vi "Datatype to Datatype String.vi"(11 "Generic Datatype":T1=enum."Bool") -> (2 "Rust String":string, 3 "String":string)   [LabVIEW 2021, in "DataTypes_CIF_U.lvlib"]
doc: "Convert generic datatypes into string names."
uses:
  DataTypes_CIF_U.lvlib
  Typedef/Generic Datatypes.ctl
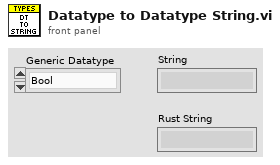
[diagram p1: front panel]
types:
  T1 = typedef "DataTypes_CIF_U.lvlib/Generic Datatypes.ctl" = enum16{"Invalid", "Bool", "U8", "I8", "U16", "I16", "U32", "I32", "U64", "I64", "Single Float", "Double Float", "String"}
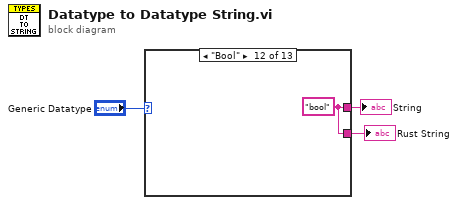
[diagram p0: block diagram]
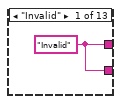
[diagram p2: hidden frame]
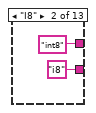
[diagram p3: hidden frame]
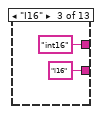
[diagram p4: hidden frame]
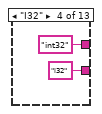
[diagram p5: hidden frame]
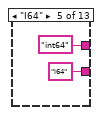
[diagram p6: hidden frame]
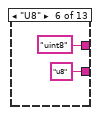
[diagram p7: hidden frame]
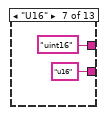
[diagram p8: hidden frame]
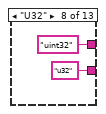
[diagram p9: hidden frame]
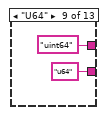
[diagram p10: hidden frame]
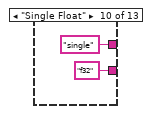
[diagram p11: hidden frame]
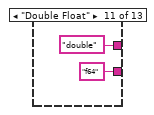
[diagram p12: hidden frame]
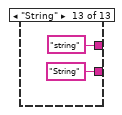
[diagram p13: hidden frame]
diagram:
  n1 = case shown="\"Bool\"" "Generic Datatype" {
    tunnel: [w4 "int8" "int16" "int32" "int64" "uint8" "uint16" "uint32" "uint64" "single" "double" w25 "string"] -> w2
    tunnel: [w4 "i8" "i16" "i32" "i64" "u8" "u16" "u32" "u64" "f32" "f64" w25 "String"] -> w1
    frame "Invalid" {
      w4 = "Invalid"
    }
    frame "I8" {
    }
    frame "I16" {
    }
    frame "I32" {
    }
    frame "I64" {
    }
    frame "U8" {
    }
    frame "U16" {
    }
    frame "U32" {
    }
    frame "U64" {
    }
    frame "Single Float" {
    }
    frame "Double Float" {
    }
    frame "Bool" {
      w25 = "bool"
    }
    frame "String" {
    }
  }
  "String" <- w2
  "Rust String" <- w1
